vi "Set Object ACL.vi"(4 "Region":T1, 6 "Version ID":string, 7 "AccessControlPolicy":T2, 8 "error in (no error)":errorcluster, 9 "Bucket":string, 10 "Object Path":string) -> (0 "error out":errorcluster, 3 "PutObjectACLResult":T5)   [LabVIEW 2015, in "LV Interface for Amazon S3.lvlib"]
doc: "This operation <B>sets the access control list (ACL) permissions for an object that already exists</B> in a bucket. (To set the ACL of an object when you put it into a bucket, use Request Parameters' ACL field of the Put Object.vi.) You <B>must have WRITE_ACP permission</B> to set the ACL of an object."
uses:
  LV Interface for Amazon S3.lvlib
  Typedefs/AMZ_S3_API_PUTObjectACLResult.ctl
  Typedefs/AMZ_S3_API_AccessControlPolicy.ctl
  Typedefs/AMZ_S3_API_Owner.ctl
  Typedefs/AMZ_S3_API_Bucket ACL Permission.ctl
  Typedefs/AMZ_S3_LocationConstraint.ctl
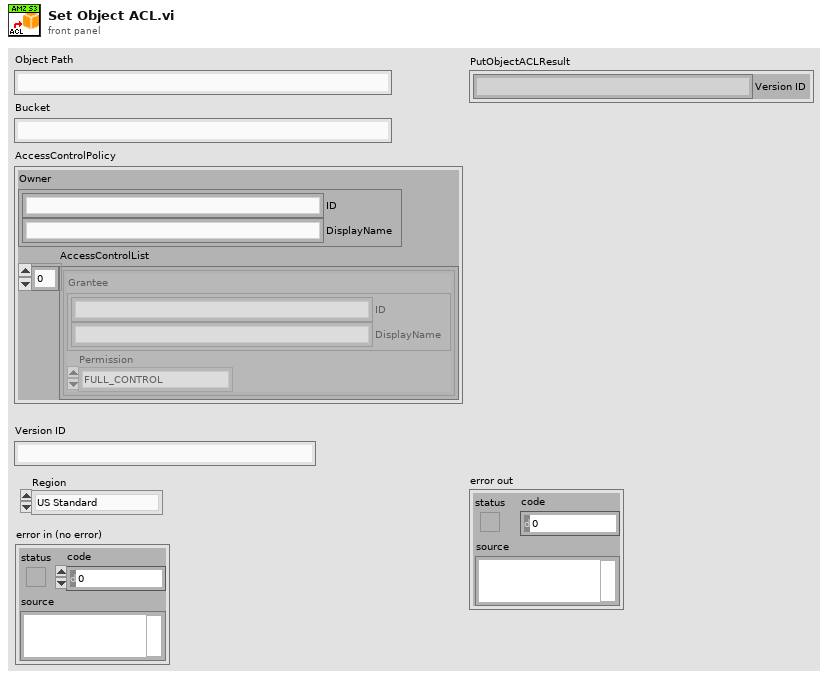
[diagram p1: front panel]
types:
  T1 = typedef "LV Interface for Amazon S3.lvlib/AMZ_S3_LocationConstraint.ctl" = enum16{"US Standard", "us-east-2", "us-west-1", "us-west-2", "ap-northeast-1", "ap-northeast-2", "ap-southeast-1", "ap-southeast-2", "ca-central-1", "eu-central-1", "eu-west-1", "eu-west-2", "sa-east-1"}
  T2 = typedef "LV Interface for Amazon S3.lvlib/AMZ_S3_API_AccessControlPolicy.ctl" = cluster{"Owner":T3, "AccessControlList":cluster{"Grantee":T3, "Permission":T4}[]}
  T3 = typedef "LV Interface for Amazon S3.lvlib/AMZ_S3_API_Owner.ctl" = cluster{"ID":string, "DisplayName":string}
  T4 = typedef "LV Interface for Amazon S3.lvlib/AMZ_S3_API_Bucket ACL Permission.ctl" = enum16{"FULL_CONTROL", "WRITE", "WRITE_ACP", "READ", "READ_ACP"}
  T5 = typedef "LV Interface for Amazon S3.lvlib/AMZ_S3_API_PUTObjectACLResult.ctl" = cluster{"Version ID":string}
  T6 = cluster{"format string":string, "Version ID":string}
  T7 = cluster{"format string":string, "Version ID":string}[]
  T8 = typedef "LV Interface for Amazon S3.lvlib/AMZ_S3_Call Results.ctl" = enum16{"Success", "UndefinedError", "AccessDenied", "AccountProblem", "AmbiguousGrantByEmailAddress", "BadDigest", "BucketAlreadyExists", "BucketAlreadyOwnedByYou", "BucketNotEmpty", "CredentialsNotSupported", "CrossLocationLoggingProhibited", "EntityTooSmall", "EntityTooLarge", "ExpiredToken", "IllegalVersioningConfigurationException", "IncompleteBody", "IncorrectNumberOfFilesInPostRequest", "InlineDataTooLarge", "InternalError", "InvalidAccessKeyId", "InvalidAddressingHeader", "InvalidArgument", "InvalidBucketName", "InvalidDigest", "InvalidLocationConstraint", "InvalidPart", "InvalidPartOrder", "InvalidPayer", "InvalidPolicyDocument", "InvalidRange", "InvalidSecurity", "InvalidSOAPRequest", "InvalidStorageClass", "InvalidTargetBucketForLogging", "InvalidToken", "InvalidURI", "KeyTooLong", "MalformedACLError", "MalformedPOSTRequest", "MalformedXML", "MaxMessageLengthExceeded", "MaxPostPreDataLengthExceededError", "MetadataTooLarge", "MethodNotAllowed", "MissingAttachment", "MissingContentLength", "MissingRequestBodyError", "MissingSecurityElement", "MissingSecurityHeader", "NoLoggingStatusForKey", "NoSuchBucket", "NoSuchKey", "NoSuchUpload", "NoSuchVersion", "NotImplemented", "NotSignedUp", "OperationAborted", "PermanentRedirect", "PreconditionFailed", "Redirect", "RequestIsNotMultiPartContent", "RequestTimeout", "RequestTimeTooSkewed", "RequestTorrentOfBucketError", "SignatureDoesNotMatch", "SlowDown", "TemporaryRedirect", "TokenRefreshRequired", "TooManyBuckets", "UnexpectedContent", "UnresolvableGrantByEmailAddress", "UserKeyMustBeSpecified", "LabVIEWError"}
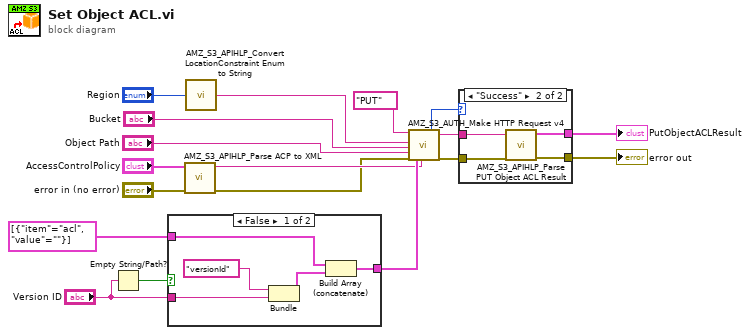
[diagram p0: block diagram]
diagram:
  n1 = Empty String/Path?(string/path="Version ID") -> (empty?=w13:bool)
  n2 = case shown="False" w13 {
    tunnel: cluster{"item":string, "value":string}[] [{"item"="acl", "value"=""}] ("request parameters") -> [w22 w24]
    tunnel: "Version ID" -> [w20 _]
    tunnel: [w19 w24] -> w8
    frame False {
      n3 = Bundle("format string"="versionId", "Version ID"=w20) -> (w21:T6)  [unwired: 1 in]
      n4 = Build Array (concatenate)(w22, w21) -> (w19:T7)
    }
    frame True {
    }
  }
  n5 = call "AMZ_S3_APIHLP_Parse ACP to XML.vi"("error in (no error)"="error in (no error)", "AccessControlPolicy"="AccessControlPolicy") -> ("error out"=w6:errorcluster, "ACP XML String"=w7:string)  [unwired: 8 in]
  n6 = call "AMZ_S3_APIHLP_Convert LocationConstraint Enum to String.vi"("Location"="Region") -> ("Location String"=w1:string)  [unwired: 4 in]
  n7 = call "AMZ_S3_AUTH_Make HTTP Request v4.vi"("HTTP-Verb"="PUT", "Region"=w1, "Bucket"="Bucket", "Object Key"="Object Path", "error in"=w6, "request parameters"=w8, "request body"=w7) -> ("Call Result"=w9:T8, "response headers"=w11:string, "error out"=w10:errorcluster)  [unwired: 9 in, 1 out]
  n8 = case shown="\"Success\"" w9 {
    tunnel: w10 -> [w25 w29]
    tunnel: w11 -> [_ w28]
    tunnel: [_ w27] -> w17
    tunnel: [w25 w26] -> w18
    frame Default {
    }
    frame "Success" {
      n9 = call "AMZ_S3_APIHLP_Parse PUT Object ACL Result.vi"("error in (no error)"=w29, "Response header"=w28) -> ("error out"=w26:errorcluster, "PutObjectACLResult"=w27:T5)  [unwired: 8 in]
    }
  }
  "error out" <- w18
  "PutObjectACLResult" <- w17
